vi "SetupPIStage.vi"() -> ()   [LabVIEW 2009]
uses:
  StageSettings.ctt
panel:
  in  "Cancel Button":bool
  in  "OK Button":bool
  in  "PI Stage Setup":T1={"channels (x, y, z)"="2,3,4", "Stage Scaling (V/µm)"=0.2} caption="Stage Setup" {"Stage Scaling (V/µm)" format="%.2f"}
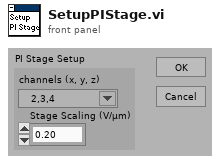
[diagram p1: front panel]
types:
  T1 = typedef "StageSettings.ctt" = cluster{"channels (x, y, z)":tag, "Stage Scaling (V/µm)":dbl}
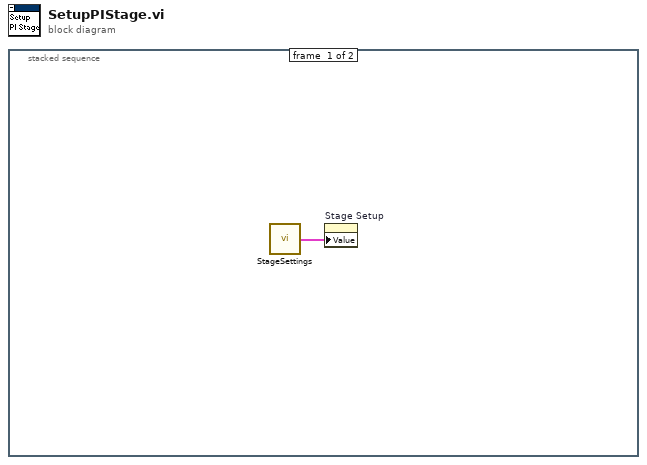
[diagram p0: block diagram]
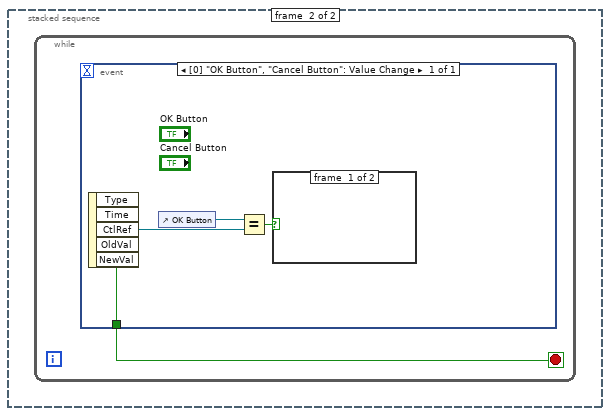
[diagram p2: hidden frame]
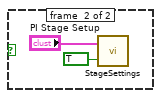
[diagram p3: hidden frame]
diagram:
  n1 = stacked-sequence {
    frame #0 {
      n2 = call "StageSettings.vi"() -> ("PI Stage Setup (output)"=w1:T1)  [unwired: 2 in]
      n3 = property on="Stage Setup" class="Clust (strict)"("Value"=w1) -> ()  [unwired: 2 in, 2 out]
    }
    frame #1 {
      n4 = while {
        stop <- w2 stop-if-true
        n5 = event shown="[0] \"OK Button\", \"Cancel Button\": Value Change" {
          selector: _ -> [_]
          dyn-events: _ -> [_]
          timeout: _ -> [_]
          tunnel: [w5] -> w2
          event [0] "OK Button", "Cancel Button": Value Change {
            n6 = event-data() -> ("CtlRef"=w6:refnum<vi>, "NewVal"=w5:bool)  [unwired: 1 in, 3 out]
            n7 = control-ref of="OK Button"() -> (w3:refnum<vi>)
            n8 = Equal?(x=w3, y=w6) -> (x = y?=w4:bool)
            n9 = case shown="True" w4 {
              frame #0 {
              }
              frame #1 {
                n10 = call "StageSettings.vi"("Get/Set"=TRUE, "PI Stage Setup (input)"="PI Stage Setup") -> ()  [unwired: 1 out]
              }
            }
          }
        }
      }
    }
  }
